vi "Adjust width for column.vi"(11 "MCListbox引用句柄":refnum<vi>) -> ()   [LabVIEW 2016]
panel:
  out "大小":i32[](array[numeric])
  out "数组":dbl[](array[numeric])
  out "转置的数组":string[][](array[string])
  out "字符串":string caption="please_change_DDD_V_30/mins bip_0.1ms_1.5"
  in  "error out":cluster{"状态":bool, "代码":i32, "源":string} caption="错误输出"
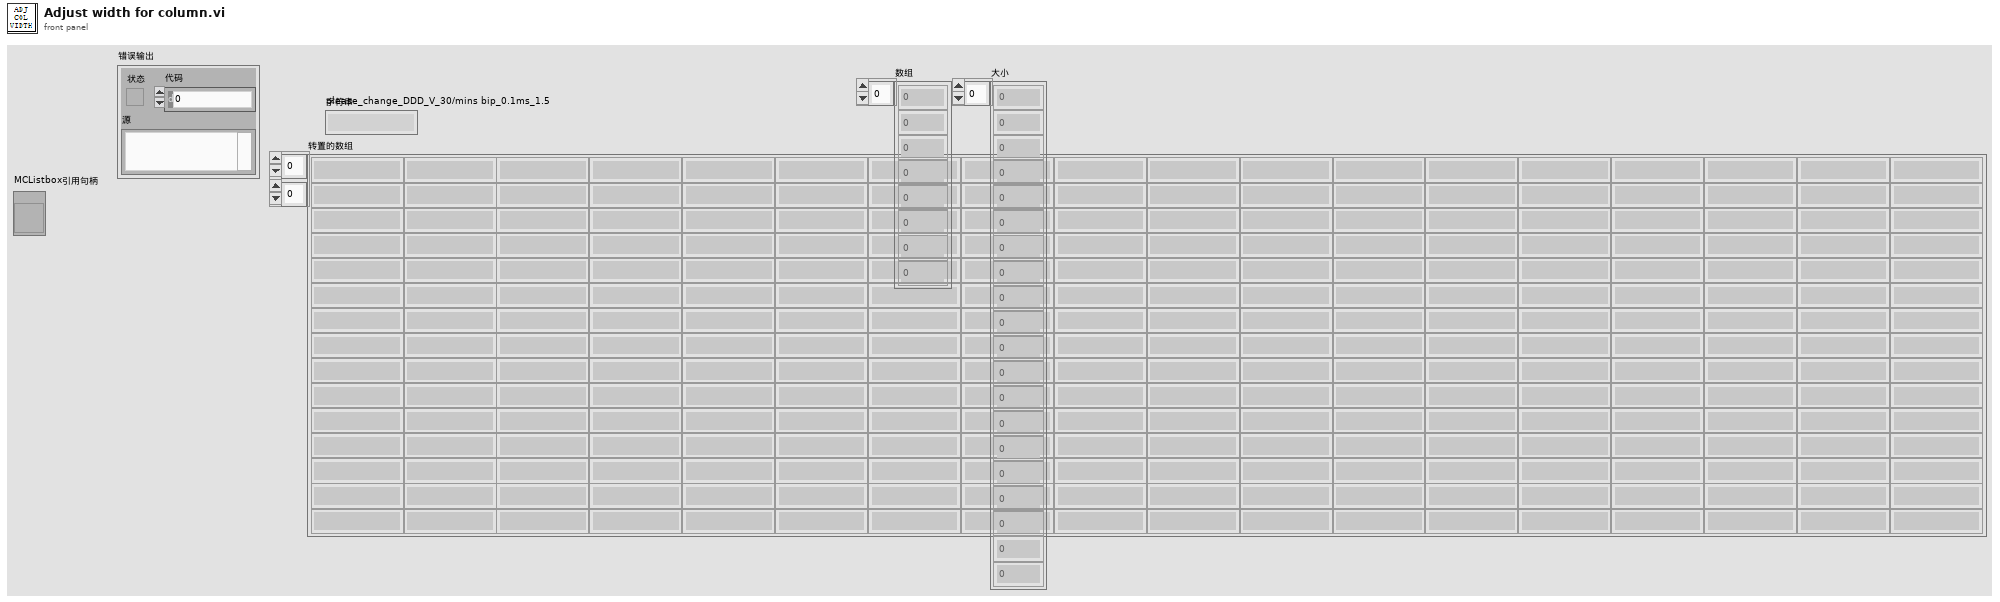
[diagram p1: front panel]
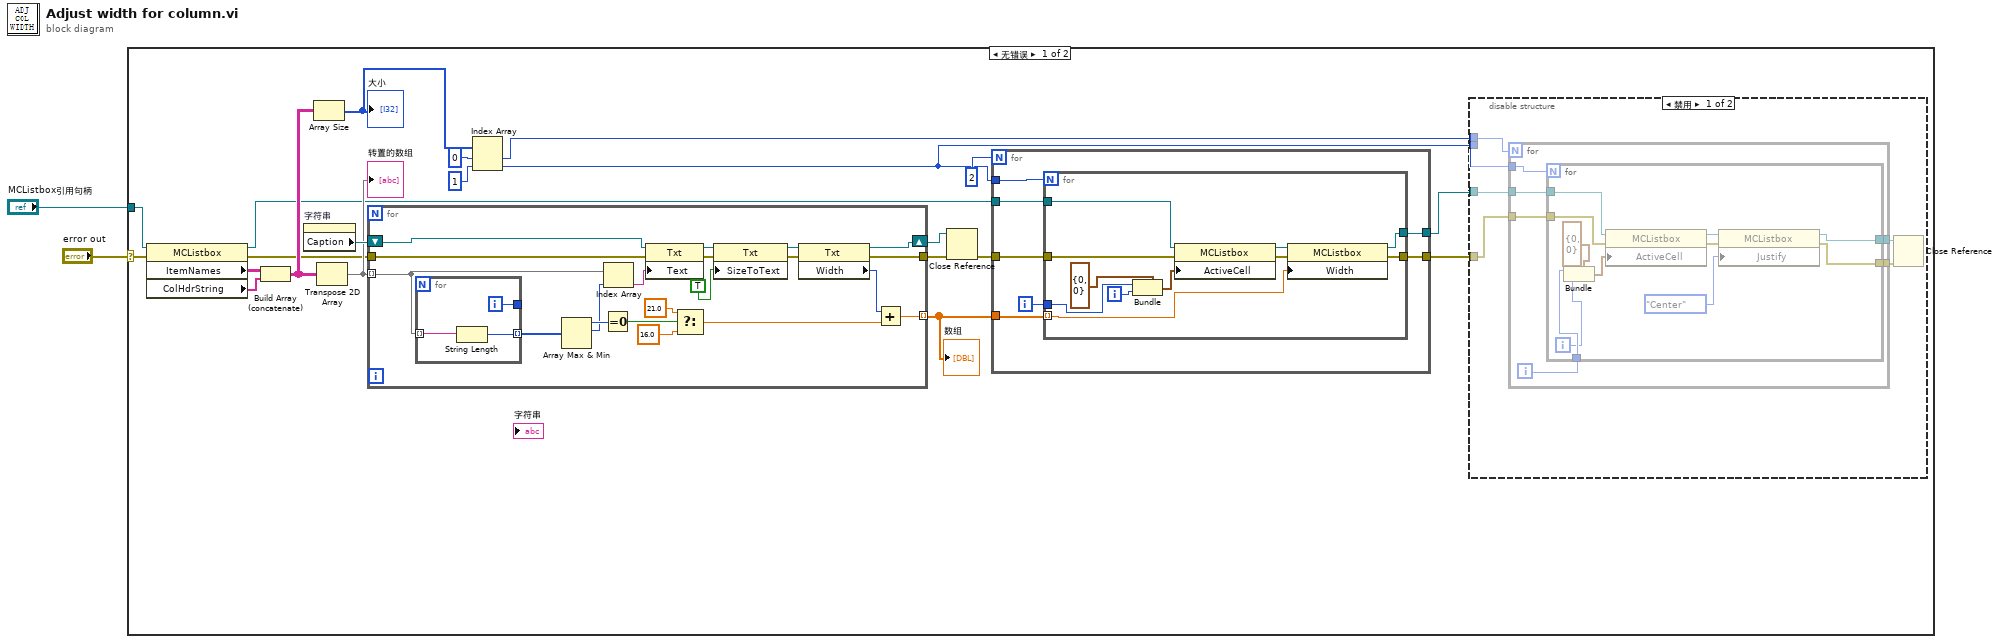
[diagram p0: block diagram]
diagram:
  n1 = case shown="无错误" "error out" {
    selector: "error out" -> [w17 _]
    tunnel: "MCListbox引用句柄" -> [w23 _]
    frame No Error {
      n2 = property class="MCListbox"(reference=w23, error in=w17) -> (reference out=w11:refnum<vi>, error out=w10:errorcluster, "ItemNames"=w22:string[][], "ColHdrString"=w21:string[])
      n3 = Build Array (concatenate)(w22, w21) -> (w16:string[][])
      n4 = property on="字符串" class="Str"() -> ("Caption"=w20:refnum<vi>)  [unwired: 2 in, 2 out]
      n5 = Array Size(array=w16) -> (size(s)=w15:i32[])
      "大小" <- w15
      n6 = Transpose 2D Array(2D array=w16) -> (transposed array=w19:string[][])
      "转置的数组" <- w19
      n7 = for {
        shift-right: [w71] -> w18
        shift-left: w20 -> [w84]
        tunnel: w19 -> [w82] mode=indexing
        tunnel: [w69] -> w12 mode=indexing
        tunnel: [w68] -> w9
        tunnel: w10 -> [w67]
        n8 = for {
          tunnel: w82 -> [w87] mode=indexing
          tunnel: [w86] -> w83 mode=indexing
          tunnel: [w85] -> _
          i -> [w85]
          n9 = String Length(string=w87) -> (length=w86:i32)
        }
        n10 = Array Max & Min(array=w83) -> (max value=w70:i32, max index (indices)=w65:i32)  [unwired: 2 out]
        n11 = Equal To 0?(x=w70) -> (x = 0?=w76:bool)
        n12 = Index Array(array=w82, index=w65) -> (element=w81:string)
        n13 = property class="Txt"(reference=w84, error in=w67, "Text"=w81) -> (reference out=w80:refnum<vi>, error out=w79:errorcluster)
        n14 = Select(t=21.0, s=w76, f=16.0) -> (s? t:f=w73:dbl)
        n15 = property class="Txt"(reference=w80, error in=w79, "SizeToText"=TRUE ("调整为文本大小？")) -> (reference out=w78:refnum<vi>, error out=w77:errorcluster)
        n16 = property class="Txt"(reference=w78, error in=w77) -> (reference out=w71:refnum<vi>, error out=w68:errorcluster, "Width"=w72:u32)
        n17 = Add(x=w72, y=w73) -> (x+y=w69:dbl)
      }
      "数组" <- w12
      n18 = Index Array(array=w15, index #1=0 ("索引"), index #2=1 ("索引")) -> (element #1=w3:i32, element #2=w4:i32)
      n19 = Close Reference(reference=w18, error in (no error)=w9) -> (error out=w8:errorcluster)
      n20 = for {
        N: 2 -> [_]
        tunnel: w12 -> [w53]
        tunnel: w4 -> [w52]
        tunnel: w11 -> [w50]
        tunnel: [w49] -> w6
        tunnel: w8 -> [w48]
        tunnel: [w47] -> w5
        i -> [w51]
        n21 = for {
          N: w52 -> [_]
          tunnel: w53 -> [w54] mode=indexing
          tunnel: w51 -> [w63]
          tunnel: w50 -> [w60]
          tunnel: [w58] -> w49
          tunnel: w48 -> [w57]
          tunnel: [w55] -> w47
          i -> [w62]
          n22 = Bundle(cluster=cluster{i32, i32} {0, 0} ("簇"), w63, w62) -> (w61:cluster{i32, i32})
          n23 = property class="MCListbox"(reference=w60, error in=w57, "ActiveCell"=w61) -> (reference out=w59:refnum<vi>, error out=w56:errorcluster)
          n24 = property class="MCListbox"(reference=w59, error in=w56, "Width"=w54) -> (reference out=w58:refnum<vi>, error out=w55:errorcluster)
        }
      }
      n25 = disable-structure shown="禁用" {
        disable-tunnel: w6 -> [w29 _]
        disable-tunnel: w5 -> [w28 _]
        disable-tunnel: w4 -> [w25 _]
        disable-tunnel: w3 -> [w24 _]
        frame Disabled {
          n26 = for {
            N: w24 -> [_]
            tunnel: w29 -> [w35]
            tunnel: w28 -> [w34]
            tunnel: [w33] -> w27
            tunnel: [w32] -> w26
            tunnel: w25 -> [w30]
            i -> [w31]
            n27 = for {
              N: w30 -> [_]
              tunnel: w35 -> [w42]
              tunnel: w34 -> [w41]
              tunnel: [w40] -> w33
              tunnel: [w39] -> w32
              tunnel: w31 -> [w37]
              i -> [w36]
              n28 = Bundle(cluster=cluster{i32, i32} {0, 0} ("簇"), w37, w36) -> (w44:cluster{i32, i32})
              n29 = property class="MCListbox"(reference=w42, error in=w41, "ActiveCell"=w44) -> (reference out=w45:refnum<vi>, error out=w46:errorcluster)
              n30 = property class="MCListbox"(reference=w45, error in=w46, "Justify"=enum16{"Left", "Center", "Right"}."Center" ("活动单元格:单元格对齐")) -> (reference out=w40:refnum<vi>, error out=w39:errorcluster)
            }
          }
          n31 = Close Reference(reference=w27, error in (no error)=w26) -> ()  [unwired: 1 out]
        }
        frame Enabled {
        }
      }
    }
    frame Error {
    }
  }
